vi "Test Pump Connection.vi"() -> ()   [LabVIEW 2018, in "VICI M6 M50 Party Mode.lvlib"]
uses:
  VICI M6 M50 Party Mode.lvlib
  <vilib>/Instr/_visa.llb/VISA Configure Serial Port (Instr).vi
panel:
  in  "stop":bool
  in  "Enum":T1(ring)
  out "read buffer 4":string
  out "Bytes at Port 5":u32
  out "String 2":string
  out "Bytes at Port 4":u32
  out "read buffer 3":string
  in  "Pump Letter":string
  out "error out":errorcluster
  out "VISA resource name out":refnum<visa-resource-name>
  in  "VISA resource name":refnum<visa-resource-name>
  in  "error in (no error)":errorcluster
  # "Copyright\\A9\\s2010\\sSchneider\\sElectric\\sMotion\\sUSA\\r\\n"
  # "Copyright© 2010 Schneider Electric Motion USA"
  # "A\\s=\\s1000000\\r\\n"
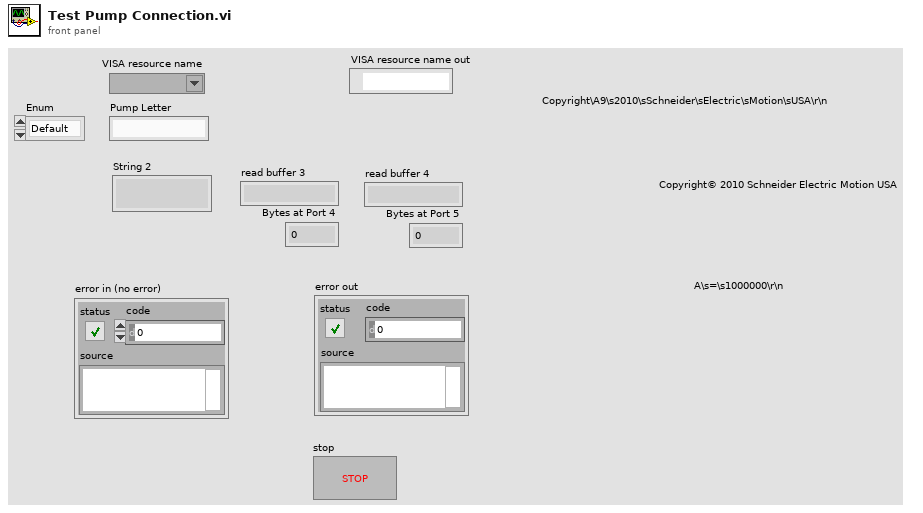
[diagram p1: front panel]
types:
  T1 = enum16{"Default", "Letter", "Save", "Party", "Test", "Single Mode", "Error Check", "Error Print"}
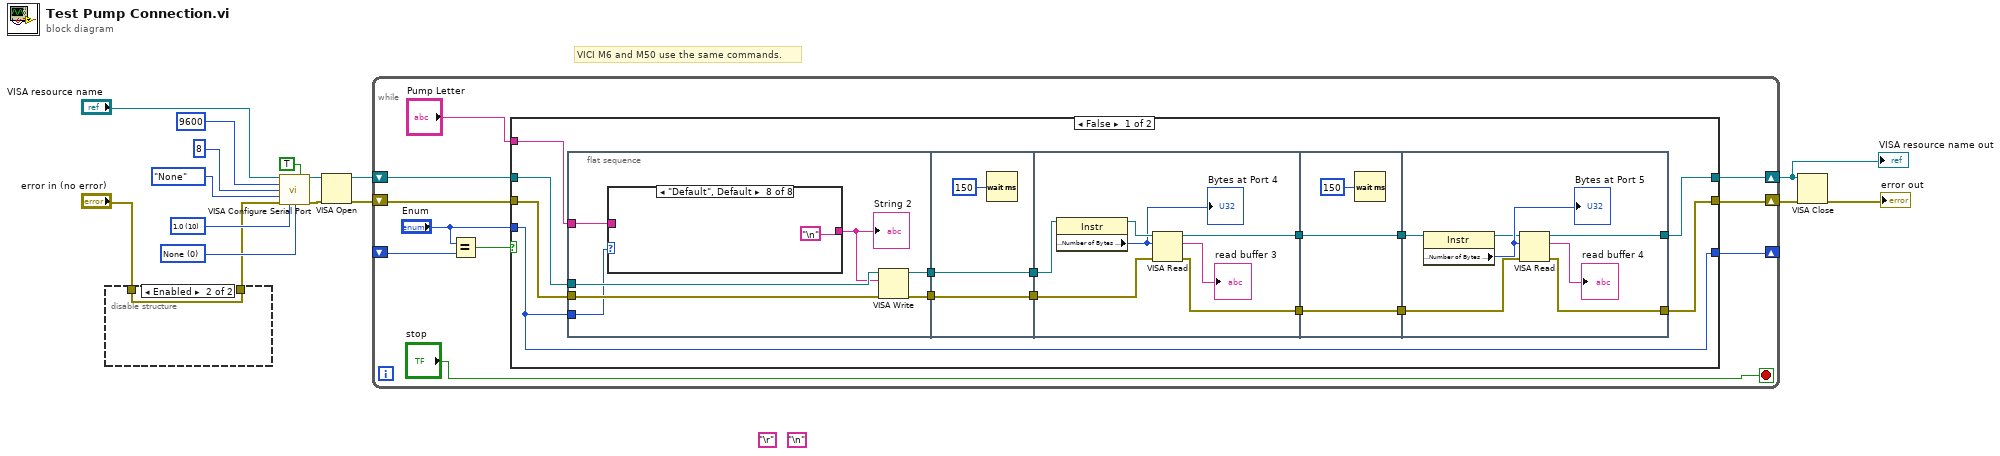
[diagram p0: block diagram]
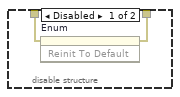
[diagram p2: hidden frame]
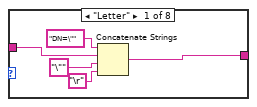
[diagram p3: hidden frame]
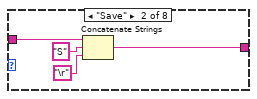
[diagram p4: hidden frame]
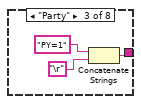
[diagram p5: hidden frame]
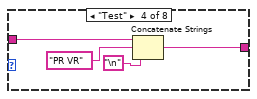
[diagram p6: hidden frame]
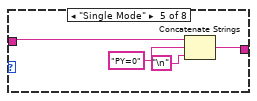
[diagram p7: hidden frame]
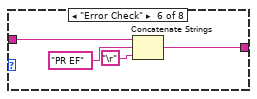
[diagram p8: hidden frame]
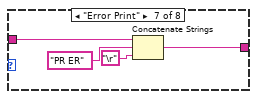
[diagram p9: hidden frame]
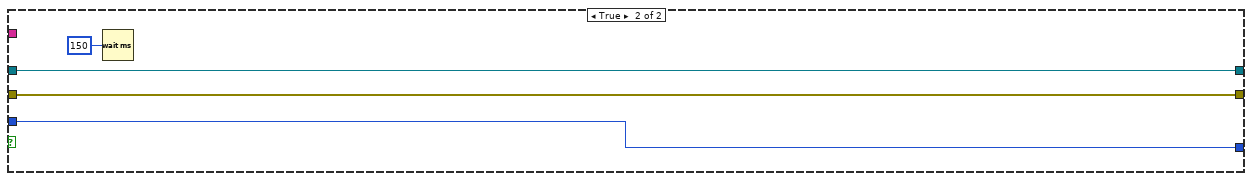
[diagram p10: hidden frame]
diagram:
  (unwired) "\r"
  (unwired) "\n"
  w9 = u16 0 items=["None", "XON/XOFF", "RTS/CTS", "XON/XOFF & RTS/CTS", "DTR/DSR", "XON/XOFF & DTR/DSR"] ("flow control (0:none)")
  w10 = u16 10 items=["1.0"=10, "1.5"=15, "2.0"=20] ("stop bits (10: 1 bit)")
  # "VICI M6 and M50 use the same commands."
  n1 = disable-structure shown="Enabled" {
    disable-tunnel: "error in (no error)" -> [w18 w19]
    disable-tunnel: [w17 w19] -> w2
    frame Disabled {
      n2 = invoke on="Enum" class="Enum (strict)" method="Reinit To Default"(error in=w18) -> (error out=w17:errorcluster)  [unwired: 2 in, 2 out]
    }
    frame Enabled {
    }
  }
  n3 = call-poly "VISA Configure Serial Port"("VISA resource name"="VISA resource name", "Enable Termination\nChar (T)"=TRUE ("Enable Termination\nChar (T)"), "baud rate (9600)"=u32 9600, "data bits (8)"=u16 8, "parity (0:none)"=enum16{"None", "Odd", "Even", "Mark", "Space"}."None", "error in (no error)"=w2, "stop bits (10: 1 bit)"=w10, "flow control (0:none)"=w9) -> ("VISA resource name out"=w15:refnum<visa-resource-name>, "error out"=w14:errorcluster)  [unwired: 6 in]
  n4 = VISA Open(error in (no error)=w14, VISA resource name=w15) -> (VISA resource name=w7:refnum<visa-resource-name>, error out=w8:errorcluster)  [unwired: 3 in]
  n5 = while {
    shift-right: [w27] -> w5
    shift-left: w8 -> [w29]
    shift-right: [w26] -> w4
    shift-left: w7 -> [w28]
    shift-right: [w24] -> _
    shift-left: _ -> [w20]
    stop <- "stop" stop-if-true
    n6 = Equal?(x="Enum", y=w20) -> (x = y?=w23:bool)
    n7 = case shown="False" w23 {
      tunnel: w29 -> [w35 w100]
      tunnel: w28 -> [w34 w101]
      tunnel: "Pump Letter" -> [w33 _]
      tunnel: [w32 w100] -> w27
      tunnel: [w31 w101] -> w26
      tunnel: "Enum" -> [w30 w102]
      tunnel: [w30 w102] -> w24
      frame False {
        n8 = flat-sequence {
          tunnel: w34 -> [w50]
          tunnel: w33 -> [w49]
          tunnel: w35 -> [w48]
          tunnel: [w47] -> w43
          tunnel: [w46] -> w42
          tunnel: w30 -> [w44]
          tunnel: [w82] -> w41
          tunnel: w43 -> [w82]
          tunnel: [w81] -> w40
          tunnel: w42 -> [w81]
          tunnel: w41 -> [w86]
          tunnel: w40 -> [w85]
          tunnel: [w84] -> w39
          tunnel: [w83] -> w38
          tunnel: w39 -> [w92]
          tunnel: [w92] -> w37
          tunnel: w38 -> [w91]
          tunnel: [w91] -> w36
          tunnel: w37 -> [w96]
          tunnel: w36 -> [w95]
          tunnel: [w94] -> w31
          tunnel: [w93] -> w32
          frame #0 {
            n9 = case shown="\"Default\", Default" w44 {
              tunnel: w49 -> [w53 w59 _ w64 w68 w71 w75 _]
              tunnel: [w52 w57 w60 w65 w69 w72 w76 "\n"] -> w45
              frame "Letter" {
                n10 = Concatenate Strings("DN=\"" ("string"), w53, "\"" ("string"), "\r") -> (w52:string)
              }
              frame "Save" {
                n11 = Concatenate Strings(w59, "S" ("string"), "\r") -> (w57:string)
              }
              frame "Party" {
                n12 = Concatenate Strings("PY=1" ("string"), "\r") -> (w60:string)
              }
              frame "Test" {
                n13 = Concatenate Strings(w64, "PR VR" ("string"), "\n") -> (w65:string)
              }
              frame "Single Mode" {
                n14 = Concatenate Strings(w68, "PY=0" ("string"), "\n") -> (w69:string)
              }
              frame "Error Check" {
                n15 = Concatenate Strings(w71, "PR EF" ("string"), "\r") -> (w72:string)
              }
              frame "Error Print" {
                n16 = Concatenate Strings(w75, "PR ER" ("string"), "\r") -> (w76:string)
              }
              frame "Default", Default {
              }
            }
            "String 2" <- w45
            n17 = VISA Write(VISA resource name=w50, write buffer=w45, error in (no error)=w48) -> (VISA resource name out=w47:refnum<visa-resource-name>, error out=w46:errorcluster)  [unwired: 1 out]
          }
          frame #1 {
            n18 = Wait (ms)(milliseconds to wait=u32 150) -> ()  [unwired: 1 out]
          }
          frame #2 {
            n19 = property class="Instr"(reference=w86) -> (reference out=w89:refnum<visa-resource-name>, "Serial Settings:Number of Bytes at Serial Port"=w88:u32)  [unwired: 1 in, 1 out]
            "Bytes at Port 4" <- w88
            n20 = VISA Read(VISA resource name=w89, byte count=w88, error in (no error)=w85) -> (VISA resource name out=w84:refnum<visa-resource-name>, read buffer=→"read buffer 3":string, error out=w83:errorcluster)  [unwired: 1 out]
          }
          frame #3 {
            n21 = Wait (ms)(milliseconds to wait=u32 150) -> ()  [unwired: 1 out]
          }
          frame #4 {
            n22 = property class="Instr"(reference=w96) -> (reference out=w97:refnum<visa-resource-name>, "Serial Settings:Number of Bytes at Serial Port"=w98:u32)  [unwired: 1 in, 1 out]
            "Bytes at Port 5" <- w98
            n23 = VISA Read(VISA resource name=w97, byte count=w98, error in (no error)=w95) -> (VISA resource name out=w94:refnum<visa-resource-name>, read buffer=→"read buffer 4":string, error out=w93:errorcluster)  [unwired: 1 out]
          }
        }
      }
      frame True {
        n24 = Wait (ms)(milliseconds to wait=u32 150) -> ()  [unwired: 1 out]
      }
    }
  }
  "VISA resource name out" <- w4
  n25 = VISA Close(VISA resource name=w4, error in (no error)=w5) -> (error out=→"error out":errorcluster)
